vi "ReadModelInfo.vi"(2 "更新量测项目序号":bool, 3 "ModelEditInfo in":T2) -> (1 "ModelEditInfo out":T2)   [LabVIEW 2014]
uses:
  <vilib>/Utility/file.llb/Read From Spreadsheet File (string).vi
  ModeEditeControl.ctl
  ModelInfo.ctl
panel:
  in  "当前产品信息":T1
  out "添加的路径":path
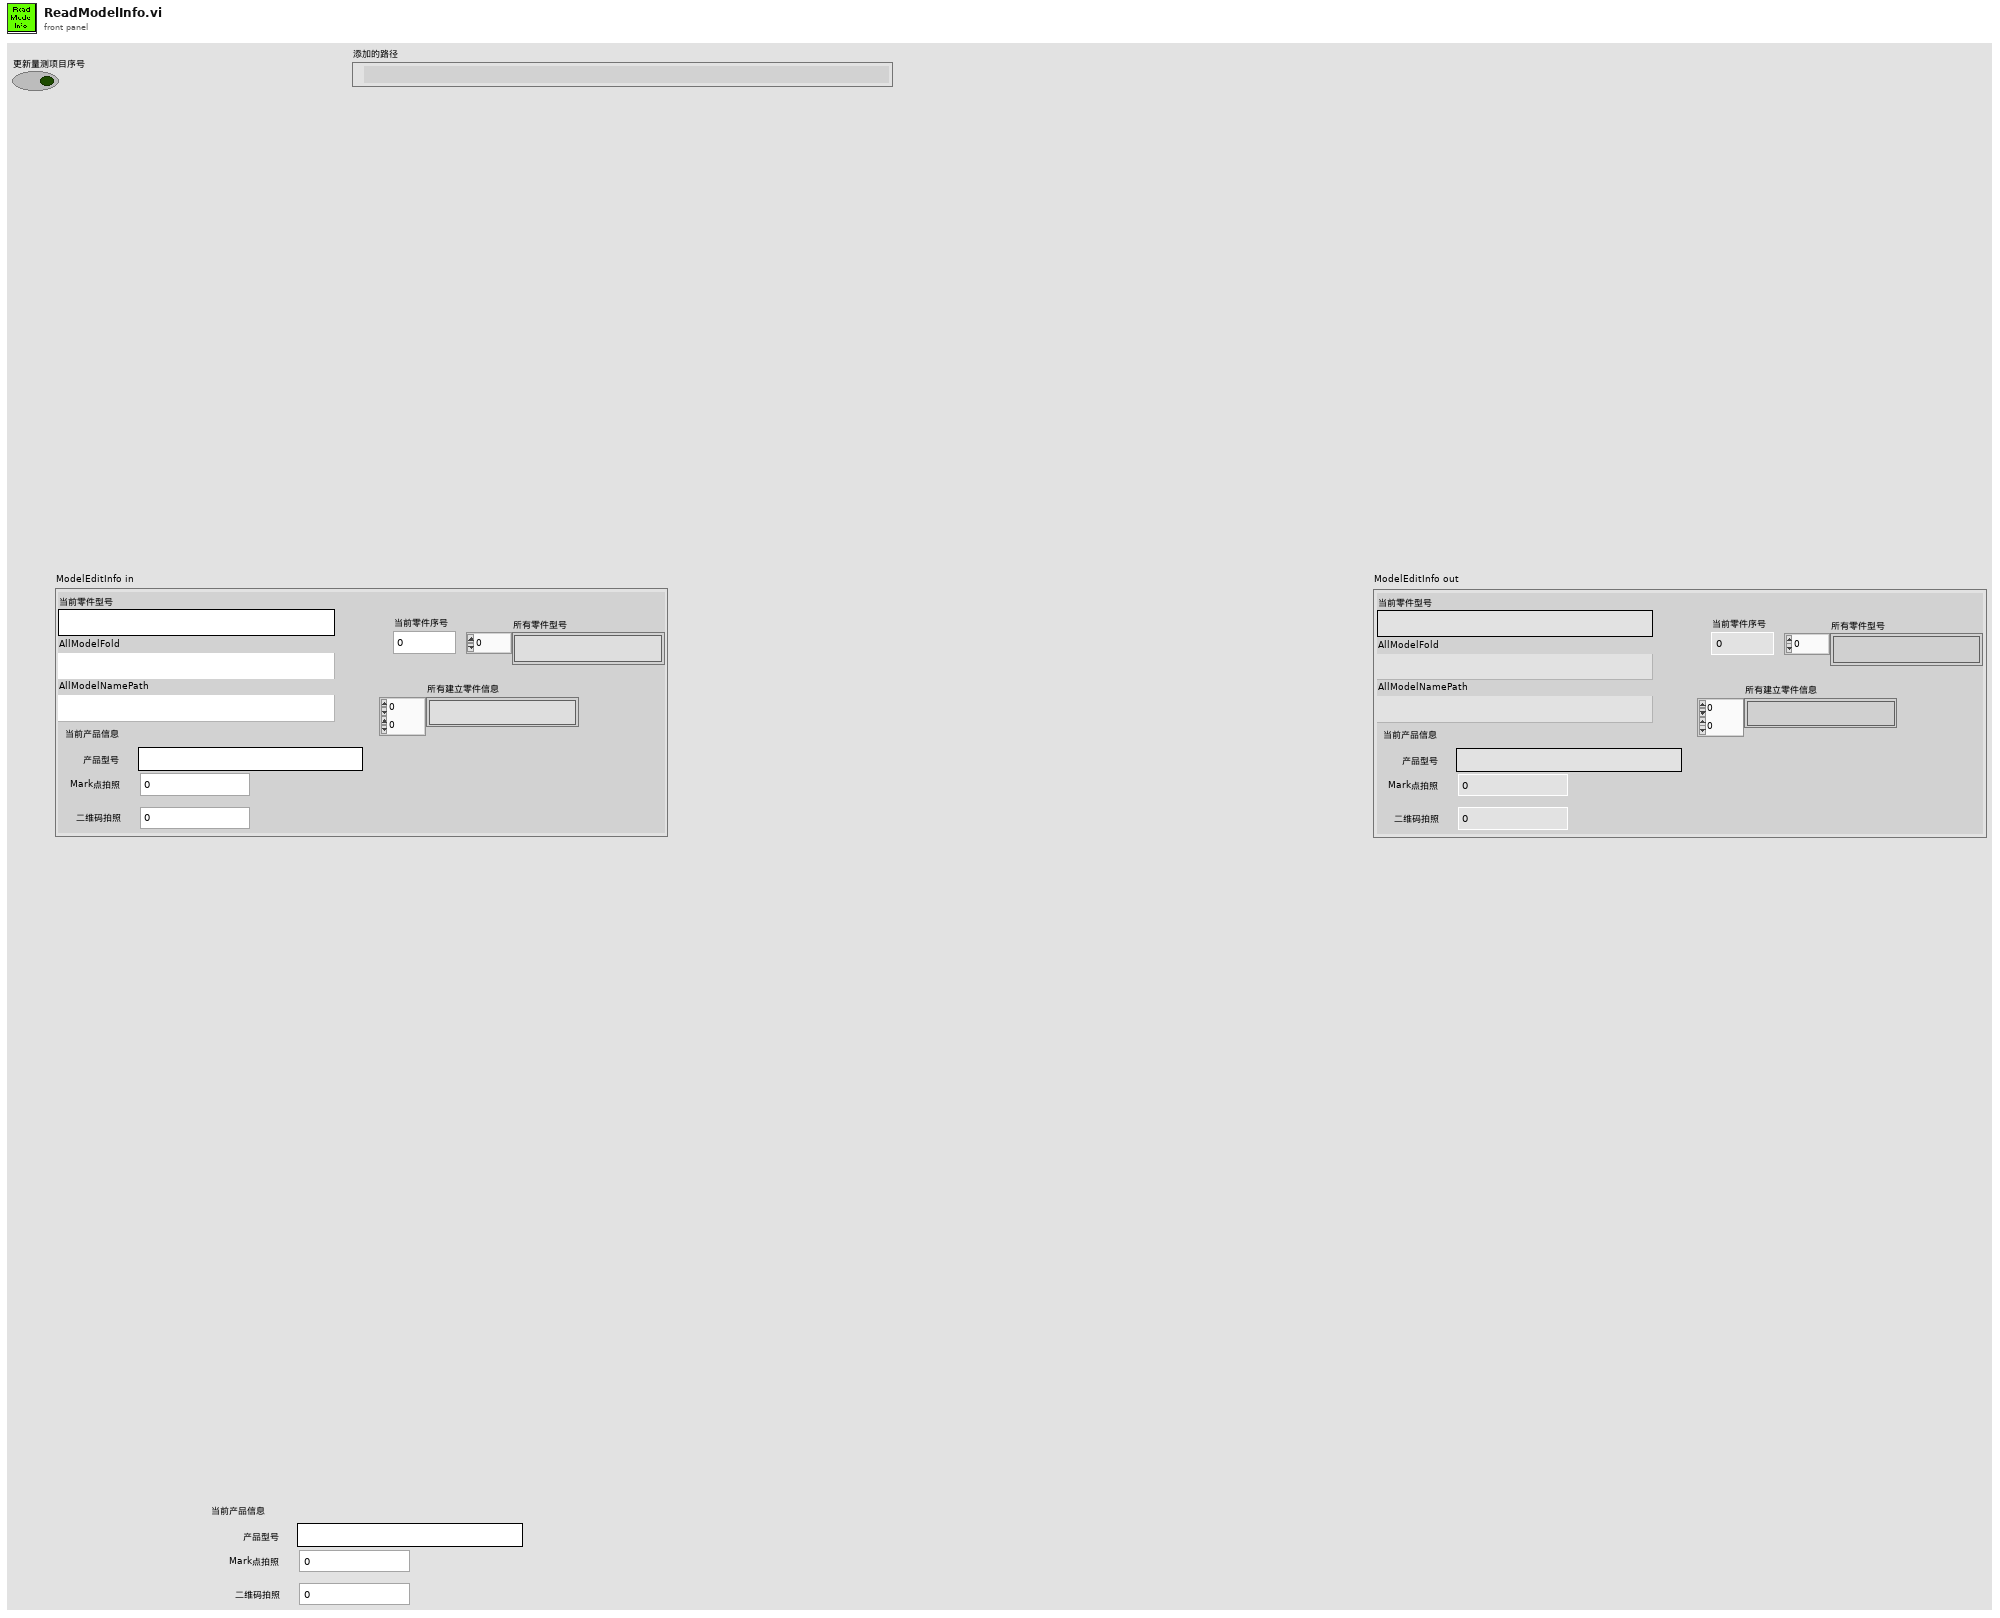
[diagram p1: front panel]
types:
  T1 = typedef "ModelInfo.ctl" = cluster{"产品型号":string, "二维码拍照":u32, "Mark点拍照":u32}
  T2 = typedef "ModeEditeControl.ctl" = cluster{"AllModelFold":path, "AllModelNamePath":path, "所有零件型号":string[], "当前零件型号":string, "所有建立零件信息":string[][], "当前零件序号":i32, "当前产品信息":T1}
  T3 = typedef "ModelInfo.ctl" = cluster{"产品型号":string, "螺丝刀型号":T4, "载具上放几片PCB":u16, "1片PCB锁几颗螺丝":u16, "CAD点位坐标文档路径":path, "托盘1螺丝型号":T5, "托盘2螺丝型号":T5, "托盘3螺丝型号":T5, "托盘4螺丝型号":T5, "托盘5螺丝型号":T5, "托盘6螺丝型号":T5, "托盘7螺丝型号":T5, "托盘8螺丝型号":T5, "托盘1螺丝锁紧程式序号":u32, "托盘2螺丝锁紧程式序号":u32, "托盘3螺丝锁紧程式序号":u32, "托盘4螺丝锁紧程式序号":u32, "托盘5螺丝锁紧程式序号":u32, "托盘6螺丝锁紧程式序号":u32, "托盘7螺丝锁紧程式序号":u32, "托盘8螺丝锁紧程式序号":u32, "预锁程式序号":u32, "复锁程式序号":u32, "复锁拍照点与Mark拍照点高度差":dbl, "取料点与P2高度差":dbl, "拍PCB孔曝光时间":u32, "取料拍螺帽曝光时间":u32, "复锁拍螺帽曝光时间":u32, "下相机曝光时间":u32}
  T4 = typedef "螺丝刀类型.ctl" = enum16{"螺丝刀1-1*3mm", "螺丝刀2-1.5*3mm", "螺丝刀3-2*3mm", "螺丝刀4-2*4mm", "螺丝刀5-2.5*4mm"}
  T5 = typedef "控件-螺丝型号.ctl" = enum16{"不供料", "一字螺丝M2.5*4", "一字螺丝M2.5*6", "一字螺丝M2.5*8", "一字螺丝M2.5*10", "一字螺丝M2.5*12", "一字螺丝M2.5*14", "一字螺丝M2.5*16", "一字螺丝M2.5*18", "一字螺丝M2.5*20", "一字螺丝M3*4", "一字螺丝M3*6", "一字螺丝M3*8", "一字螺丝M3*10", "一字螺丝M3*12", "一字螺丝M3*14", "一字螺丝M3*16", "一字螺丝M3*18", "一字螺丝M3*20", "一字螺丝M4*6", "一字螺丝M4*8", "一字螺丝M4*10", "一字螺丝M4*12", "一字螺丝M4*14", "一字螺丝M4*16", "一字螺丝M4*18", "一字螺丝M4*20", "十字螺丝M2.5*4", "十字螺丝M2.5*6", "十字螺丝M2.5*8", "十字螺丝M2.5*10", "十字螺丝M2.5*12", "十字螺丝M2.5*14", "十字螺丝M2.5*16", "十字螺丝M2.5*18", "十字螺丝M2.5*20", "十字螺丝M3*4", "十字螺丝M3*6", "十字螺丝M3*8", "十字螺丝M3*10", "十字螺丝M3*12", "十字螺丝M3*14", "十字螺丝M3*16", "十字螺丝M3*18", "十字螺丝M3*20", "十字螺丝M4*6", "十字螺丝M4*8", "十字螺丝M4*10", "十字螺丝M4*12", "十字螺丝M4*14", "十字螺丝M4*16", "十字螺丝M4*18", "十字螺丝M4*20"}
  T6 = typedef "ModeEditeControl.ctl" = cluster{"Root":path, "AllModelFold":path, "AllModelNamePath":path, "所有零件型号":string[], "当前零件型号":string, "所有建立零件信息":string[][], "当前零件序号":i32, "当前产品所有点位信息":cluster{"当前点位序号":i32, "点位信息路径":path, "CAD点位坐标路径":path, "点位信息表":string[][], "当前点位信息":T7, "CAD图纸点位个数":i32}, "当前产品信息":T3, "所有螺丝和垫片型号Path":path, "Mark拍照点坐标":T11[][], "自动锁螺丝: PCB孔拍照点-多片PCB(去除未勾选的)":T11[], "8个供料盘是否供料-1PCB(去除未勾选的)":bool[], "8个供料盘是否拍照取料":bool[], "自动锁螺丝: 1PCB每颗螺丝来自哪个供料盘U8(去除未勾选的)":u8[], "自动锁螺丝: 1PCB每颗螺丝拧紧程式编号U8(去除未勾选的)":u8[], "4个预锁程式+4个复锁程式编号U8":u8[], "自动锁螺丝: 锁螺丝相对拍照时旋转角度-多片PCB(去除未勾选的)":i32[], "自动锁螺丝: 点位补偿值-多片PCB(去除未勾选的)":T8[], "1PCB上自动锁螺丝个数(去除未勾选的)":i32, "自动锁螺丝: 放料点相对拍照点高度差-多片PCB(去除未勾选的)":dbl[], "8个供料盘是否供料(包括未勾选的)":bool[], "已勾选的自动锁螺丝点位供料盘设定错误":bool, "自动锁螺丝: 复锁拍照点-多片PCB(去除未勾选的)":T11[][], "自动锁螺丝: 1PCB每颗螺丝外径*10(去除未勾选的)":u32[], "拧紧程式参数":cluster{"所有拧紧程式参数表路径":path, "所有拧紧程式参数表":string[][], "自动锁螺丝: 每个托盘螺丝拧紧程式参数":T12[], "自动锁螺丝: 预锁复锁拧紧程式参数":T12[], "所有拧紧程式参数表当前行":i32}, "已勾选的自动锁螺丝点位拧紧程式序号设定错误":bool}
  T7 = typedef "锁附点位信息.ctl" = cluster{"点位名称":string, "点位坐标(图纸)":T8, "点位坐标(实际)":T9, "补偿值":T8, "锁附时机械手角度":T10, "放料点相对Mark\n拍照点高度差":dbl, "选择螺丝托盘":enum32{"托盘1", "托盘2", "托盘3", "托盘4", "托盘5", "托盘6", "托盘7", "托盘8"}, "拧紧程式序号":u16, "预锁程式序号":u16, "复锁程式序号":u16, "自动锁螺丝":bool}
  T8 = typedef "XYZPos.ctl" = cluster{"X":dbl, "Y":dbl, "Z":dbl}
  T9 = typedef "XYZRPos.ctl" = cluster{"X":dbl, "Y":dbl, "Z":dbl, "R":dbl}
  T10 = typedef "锁附时机械手角度.ctl" = enum16{"0度", "顺时针90度", "顺时针180度", "逆时针90度", "逆时针180度"}
  T11 = typedef "XYZRPos+左右手.ctl" = cluster{"坐标":T9, "左右手":dbl}
  T12 = typedef "控件-拧紧程式参数.ctl" = cluster{"螺距":dbl, "入牙段转速":dbl, "入牙段转角":dbl, "快速段转速":dbl, "快速段转角":dbl, "快速段Z补偿":dbl, "拧紧转速":dbl}
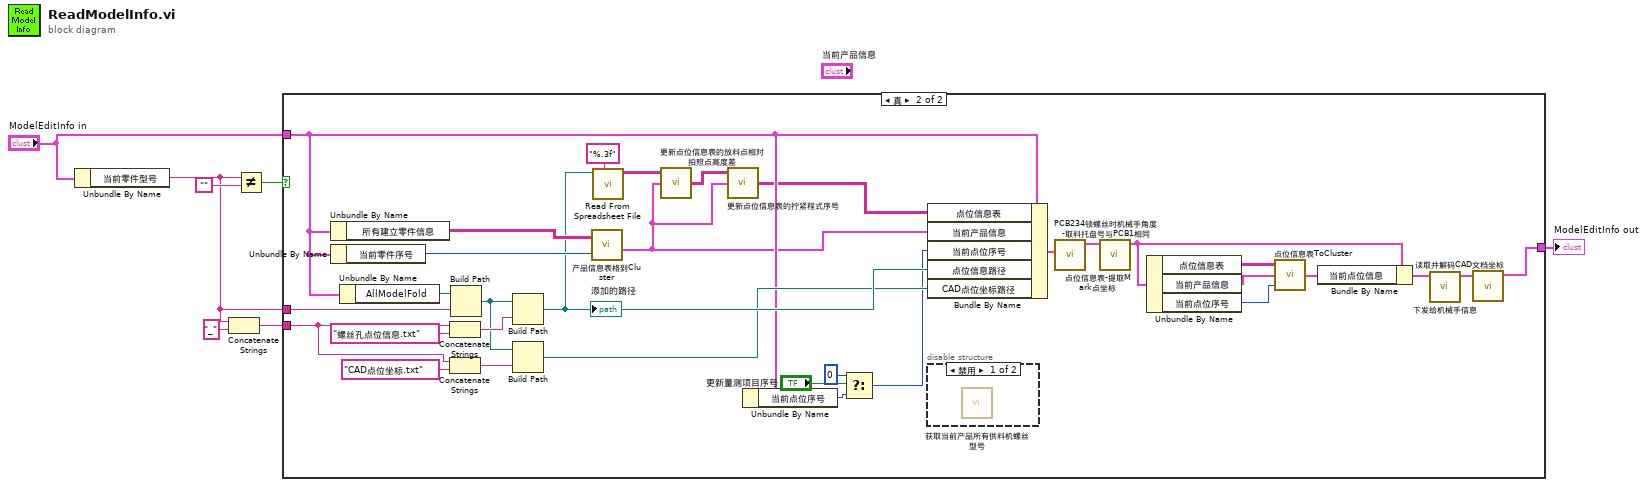
[diagram p0: block diagram]
diagram:
  n1 = Unbundle By Name("ModelEditInfo in") -> ("当前零件型号"=w3:string)
  n2 = Concatenate Strings(w3, "_" ("字符串")) -> (w1:string)
  n3 = Not Equal?(x=w3, y="") -> (x != y?=w7:bool)
  n4 = case shown="真" w7 {
    tunnel: "ModelEditInfo in" -> [w8 w23]
    tunnel: [w8 w25] -> w5
    tunnel: w3 -> [_ w39]
    tunnel: w1 -> [_ w30]
    frame False {
    }
    frame True {
      n5 = Unbundle By Name(w23) -> ("所有建立零件信息"=w36:string[][])
      n6 = Unbundle By Name(w23) -> ("当前零件序号"=w35:i32)
      n7 = Unbundle By Name(w23) -> ("AllModelFold"=w40:path)
      n8 = Concatenate Strings(w30, "螺丝孔点位信息.txt" ("名称或相对路径")) -> (w37:string)
      n9 = Concatenate Strings(w30, "CAD点位坐标.txt" ("名称或相对路径")) -> (w27:string)
      n10 = Build Path(base path=w40, name or relative path=w39) -> (appended path=w28:path)
      n11 = Build Path(base path=w28, name or relative path=w37) -> (appended path=w29:path)
      "添加的路径" <- w29
      n12 = Build Path(base path=w28, name or relative path=w27) -> (appended path=w26:path)
      n13 = call "产品信息表格到Cluster.vi"("Row"=w35, "已建立量测零件信息"=w36) -> ("零件信息"=w17:T3)
      n14 = call-poly <vilib>:"Read From Spreadsheet File.vi"("format (%s)"="%.3f", "file path (dialog if empty)"=w29) -> ("all rows"=w22:string[][])  [unwired: 5 in, 4 out]
      n15 = call "更新点位信息表的放料点相对拍照点高度差.vi"("当前产品信息"=w17, "锁螺丝点位信息表"=w22) -> ("更新放料点与拍照点高度差后的锁附点位信息表"=w21:string[][])  [unwired: 1 in]
      n16 = call "更新点位信息表的拧紧程式序号.vi"("当前产品信息"=w17, "锁螺丝点位信息表"=w21) -> ("更新拧紧程式序号后的锁附点位信息表"=w20:string[][])  [unwired: 1 in]
      n17 = Unbundle By Name(w23) -> ("当前点位序号"=w33:i32)
      n18 = Select(t=0 ("当前量测零件信息.当前量测项目序号"), s="更新量测项目序号", f=w33) -> (s? t:f=w16:i32)
      n19 = Bundle By Name(cluster=w23, "点位信息表"=w20, "当前产品信息"=w17, "当前点位序号"=w16, "点位信息路径"=w29, "CAD点位坐标路径"=w26) -> (w19:T2)
      n20 = disable-structure shown="禁用" {
        frame Disabled {
          n21 = call "获取当前产品所有供料机螺丝型号.vi"() -> ()  [unwired: 11 in, 1 out]
        }
        frame Enabled {
        }
      }
      n22 = call "PCB234锁螺丝时机械手角度-取料托盘号与PCB1相同.vi"("ModelEditInfo输入"=w19) -> ("ModelEditInfo out"=w14:T6)  [unwired: 9 in, 1 out]
      n23 = call "点位信息表-提取Mark点坐标.vi"("ModelEditInfo in"=w14) -> ("ModelEditInfo输出"=w13:T2)  [unwired: 10 in]
      n24 = Unbundle By Name(w13) -> ("点位信息表"=w12:string[][], "当前产品信息"=w11:T1, "当前点位序号"=w10:i32)
      n25 = call "点位信息表ToCluster.vi"("Row"=w10, "当前产品信息"=w11, "锁附点位信息表"=w12) -> ("锁附点位信息"=w15:T7)
      n26 = Bundle By Name(cluster=w13, "当前点位信息"=w15) -> (w18:T2)
      n27 = call "下发给机械手信息.vi"("ModelEditInfo"=w18) -> ("ModelEditInfo out"=w9:T2)  [unwired: 10 in]
      n28 = call "读取并解码CAD文档坐标.vi"("ModelEditInfo"=w9) -> ("ModelEditInfo 输出"=w25:T2)  [unwired: 10 in]
    }
  }
  "ModelEditInfo out" <- w5
